vi "Defer Panel Updates.vi"(8 "error in (no error)":errorcluster, 10 "Defer Panel Updates [T]":bool=TRUE, 11 "VI Ref":refnum<vi>) -> (0 "error out":errorcluster, 3 "VI Ref Out":refnum<vi>)   [LabVIEW 2023]
doc: "Defers updates on calling VIs panel, or releases the deferment.\n\nIf VI ref not passed in, go up call chain to find first open panel and defer on that."
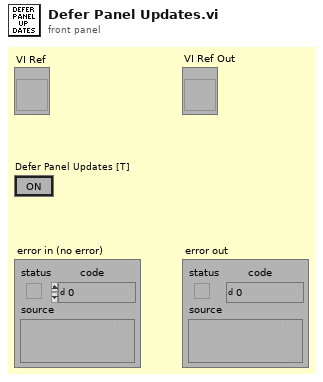
[diagram p1: front panel]
types:
  T1 = enum32{"Invalid", "Standard", "Closed", "Hidden", "Minimized", "Maximized"}
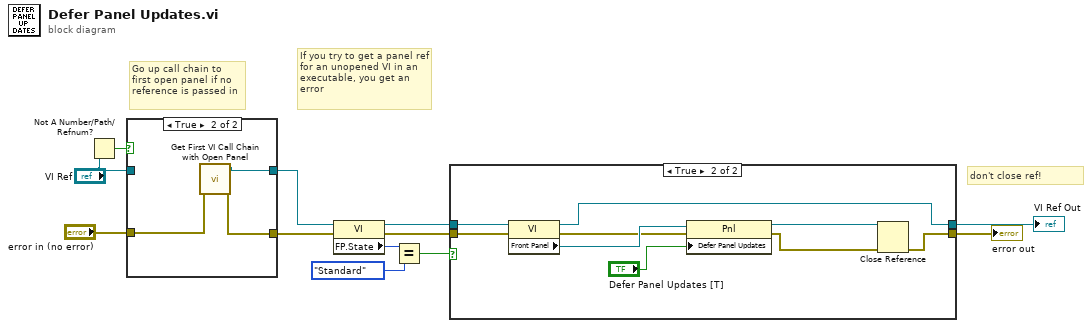
[diagram p0: block diagram]
diagram:
  # "don't close ref!"
  # "Go up call chain to first open panel if no reference is passed in"
  # "If you try to get a panel ref for an unopened VI in an executable, you get an error"
  n1 = Not A Number/Path/Refnum?(number/path/refnum="VI Ref") -> (NaN/Path/Refnum?=w12:bool)
  n2 = case shown="True" w12 {
    tunnel: [w14 w17] -> w2
    tunnel: "VI Ref" -> [w14 _]
    tunnel: "error in (no error)" -> [w13 w16]
    tunnel: [w13 w15] -> w3
    frame False {
    }
    frame True {
      n3 = call "Get First VI Call Chain with Open Panel.vi"("error in (no error)"=w16) -> ("error out"=w15:errorcluster, "vi reference"=w17:refnum<vi>)  [unwired: 8 in, 1 out]
    }
  }
  n4 = property class="VI"(reference=w2, error in=w3) -> (reference out=w1:refnum<vi>, error out=w8:errorcluster, "FP.State"=w11:T1)
  n5 = Equal?(x=w11, y=T1."Standard" ("Front Panel Window:State")) -> (x = y?=w7:bool)
  n6 = case shown="True" w7 {
    tunnel: [w19 w21] -> w6
    tunnel: w8 -> [w19 w28]
    tunnel: [w18 w20] -> w5
    tunnel: w1 -> [w18 w22]
    frame False {
    }
    frame True {
      n7 = property class="VI"(reference=w22, error in=w28) -> (reference out=w20:refnum<vi>, error out=w25:errorcluster, "Front Panel"=w27:refnum<vi>)
      n8 = property class="Pnl"(reference=w27, error in=w25, "Defer Panel Updates"="Defer Panel Updates [T]") -> (reference out=w26:refnum<vi>, error out=w23:errorcluster)
      n9 = Close Reference(reference=w26, error in (no error)=w23) -> (error out=w21:errorcluster)
    }
  }
  "error out" <- w6
  "VI Ref Out" <- w5
